vi "Set Colleague Name.vi"(8 "error in (no error)":errorcluster caption="错误输入（无错误）", 10 "同事名称":string, 11 "同事（抽象）输入":refnum<class "Colleague.lvclass">) -> (0 "error out":errorcluster caption="错误输出", 3 "同事（抽象）输出":refnum<class "Colleague.lvclass">)   [LabVIEW 2011, in "Colleague.lvclass"]
uses:
  Colleague.lvclass
  Colleague.lvclass/Colleague.ctl
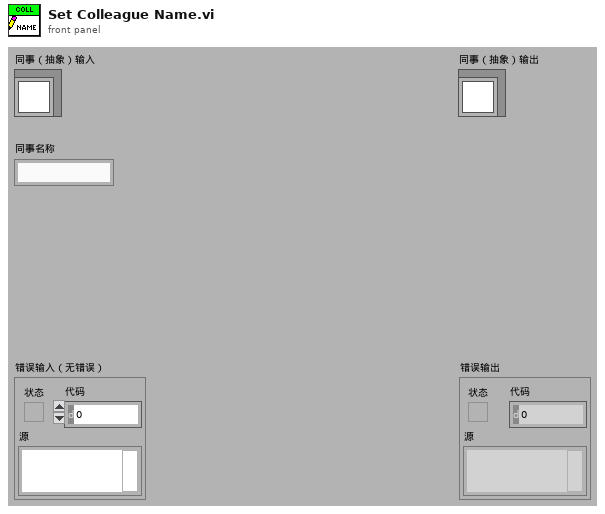
[diagram p1: front panel]
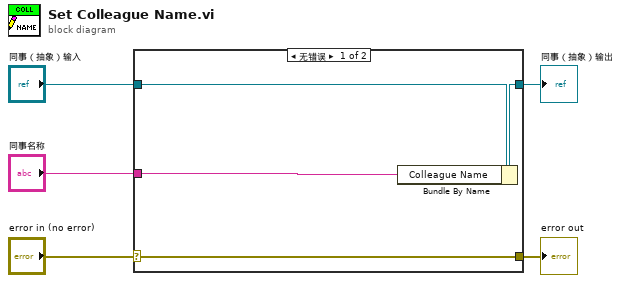
[diagram p0: block diagram]
diagram:
  n1 = case shown="无错误" "error in (no error)" {
    selector: "error in (no error)" -> [w9 w10]
    tunnel: [w9 w10] -> w4
    tunnel: [w7 w11] -> w2
    tunnel: "同事（抽象）输入" -> [w8 w11]
    tunnel: "同事名称" -> [w6 _]
    frame No Error {
      n2 = Bundle By Name(cluster=w8, "Colleague Name"=w6) -> (w7:refnum<class "Colleague.lvclass">)
    }
    frame Error {
    }
  }
  "error out" <- w4
  "同事（抽象）输出" <- w2
